vi "Ring.vi"(8 "error in (no error)":errorcluster, 11 "CellPhone in":refnum<class "CellPhone.lvclass">) -> (0 "error out":errorcluster, 3 "CellPhone out":refnum<class "CellPhone.lvclass">)   [LabVIEW 2009, in "CellPhone.lvclass"]
doc: "Causes the Cellphone to ring."
uses:
  CellPhone.lvclass
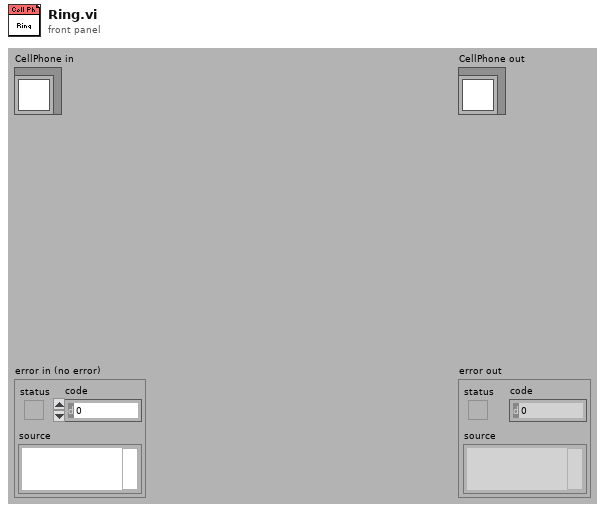
[diagram p1: front panel]
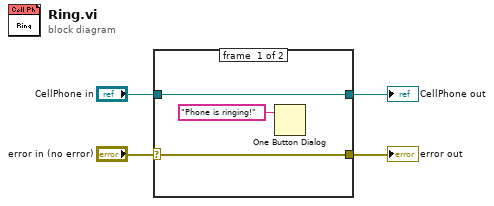
[diagram p0: block diagram]
diagram:
  n1 = case shown="No Error" "error in (no error)" {
    selector: "error in (no error)" -> [w6 w9]
    tunnel: [w6 w9] -> w3
    tunnel: [w7 w8] -> w1
    tunnel: "CellPhone in" -> [w7 w8]
    frame #0 {
      n2 = One Button Dialog(message="Phone is ringing!") -> ()  [unwired: 1 in, 1 out]
    }
    frame #1 {
    }
  }
  "error out" <- w3
  "CellPhone out" <- w1
